vi "SwerveLoadOffsets.vi"(8 "error in (no error)":errorcluster) -> (0 "error out":errorcluster)   [LabVIEW 2016, in "Team900SwerveDrive.lvlib"]
uses:
  Team900SwerveDrive.lvlib
  <vilib>/Utility/config.llb/Read Key (Double).vi
  SwerveGlobalData.vi
  <vilib>/Utility/config.llb/NI_LVConfig.lvlib
panel:
  out "Offsets":dbl[](array[numeric])
  # "Loads the offsets for the four wheels from the config file"
  # "Thought: SaveOffsets.vi is unnecessary, but a VI that\nchecks if there is a config file and creates one with\nthe correct keys would be a good idea (see\nOpenConfig.vi in Team900-VI's)"
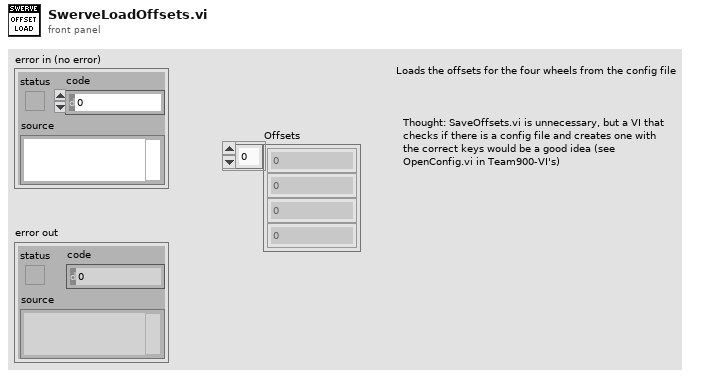
[diagram p1: front panel]
types:
  T1 = typedef "NI_LVConfig.lvlib/Config Data RefNum.ctl" = refnum<k1>
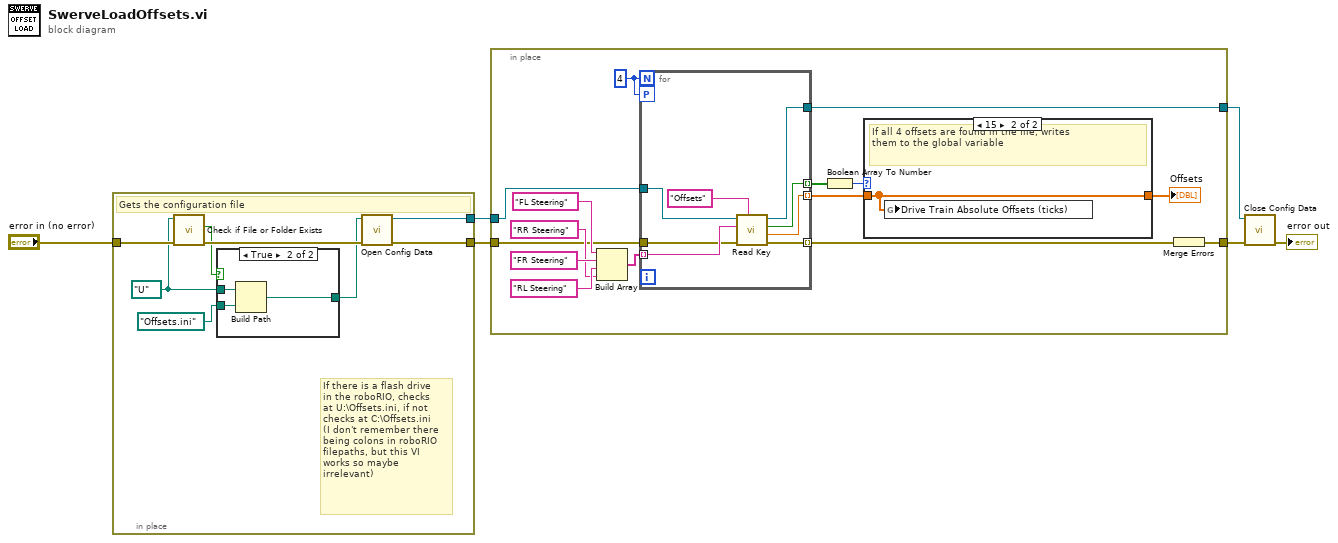
[diagram p0: block diagram]
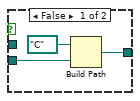
[diagram p2: hidden frame]
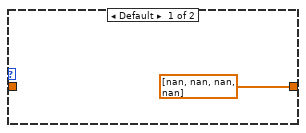
[diagram p3: hidden frame]
diagram:
  n1 = in-place {
    in-place-border: "error in (no error)" -> [w14]
    in-place-border: [w12] -> w5
    in-place-border: [w11] -> w4
    w7 = path "U:/" ("base path")
    # "If there is a flash drive\nin the roboRIO, checks\nat U:\\Offsets.ini, if not \nchecks at C:\\Offsets.ini\n(I don't remember there\nbeing colons in roboRIO\nfilepaths, but this VI\nworks so maybe \nirrelevant)"
    # "Gets the configuration file"
    n2 = call <vilib>:"Check if File or Folder Exists.vi"("error in (no error)"=w14, "path"=w7) -> ("error out"=w13:errorcluster, "file or folder exists?"=w8:bool)  [unwired: 7 in, 1 out]
    n3 = case shown="True" w8 {
      tunnel: path "Offsets.ini" ("default name") -> [w17 w18]
      tunnel: [w16 w19] -> w10
      tunnel: w7 -> [_ w20]
      frame False {
        n4 = Build Path(base path=path "C:/", name or relative path=w17) -> (appended path=w16:path)
      }
      frame True {
        n5 = Build Path(base path=w20, name or relative path=w18) -> (appended path=w19:path)
      }
    }
    n6 = call <vilib>:"Open Config Data.vi"("error in (no error)"=w13, "configuration file path"=w10) -> ("error out"=w12:errorcluster, "refnum"=w11:T1)  [unwired: 1 in, 7 out]
  }
  n7 = in-place {
    in-place-border: w5 -> [w25]
    in-place-border: [w22] -> w3
    in-place-border: w4 -> [w24]
    in-place-border: [w23] -> w2
    w35 = 4
    n8 = Build Array("FL Steering", "FR Steering" ("element"), "RL Steering" ("element"), "RR Steering" ("element")) -> (w30:string[])
    n9 = for {
      N: w35 -> [_]
      workers-P: w35 -> [_]
      tunnel: w30 -> [w45] mode=indexing
      tunnel: w24 -> [w44]
      tunnel: [w43] -> w28 mode=indexing
      tunnel: w25 -> [w42]
      tunnel: [w41] -> w29 mode=indexing
      tunnel: [w40] -> w27 mode=indexing
      tunnel: [w39] -> w23
      n10 = call-poly <vilib>:"Read Key.vi"("section"="Offsets", "error in (no error)"=w42, "key"=w45, "refnum"=w44) -> ("error out"=w41:errorcluster, "value"=w43:dbl, "found?"=w40:bool, "refnum out"=w39:T1)  [unwired: 4 in]
    }
    n11 = Boolean Array To Number(Boolean array=w27) -> (number=w26:u32)
    n12 = case shown="15" w26 {
      tunnel: w28 -> [_ w37]
      tunnel: [dbl[] [nan, nan, nan, nan] w37] -> w21
      frame Default {
      }
      frame 15 {
        # "If all 4 offsets are found in the file, writes\nthem to the global variable"
        n13 = global write "SwerveGlobalData.vi" "Drive Train Absolute Offsets (ticks)"(w37) -> ()
      }
    }
    "Offsets" <- w21
    n14 = Merge Errors(w29) -> (w22:errorcluster)
  }
  n15 = call <vilib>:"Close Config Data.vi"("error in (no error)"=w3, "refnum"=w2) -> ("error out"=→"error out":errorcluster)  [unwired: 8 in, 1 out]
